vi "NonRobotDebugger.vi"() -> ()   [LabVIEW 2012]
uses:
  <vilib>/Utility/inputDevices.llb/joystickAcquire.vi
panel:
  out "Output Right":dbl(slide) scale=-1.0..1.0
  out "Output Left":dbl(slide) scale=-1.0..1.0
  out "X axis":dbl(slide) scale=-1.0..1.0
  out "Y axis":dbl(slide) scale=-1.0..1.0
  out "Throttle":dbl
  out "Steering":dbl
  out "Left Side Motors":dbl
  out "Right Side Motors":dbl
  in  "Gear":bool
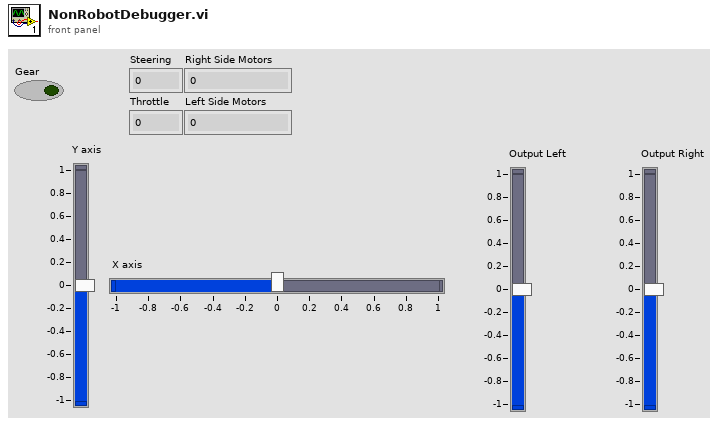
[diagram p1: front panel]
types:
  T1 = cluster{"X axis":i32, "Y axis":i32, "Z axis":i32, "X axis rotation":i32, "Y axis rotation":i32, "Z axis rotation":i32, "U axis":i32, "V axis":i32}
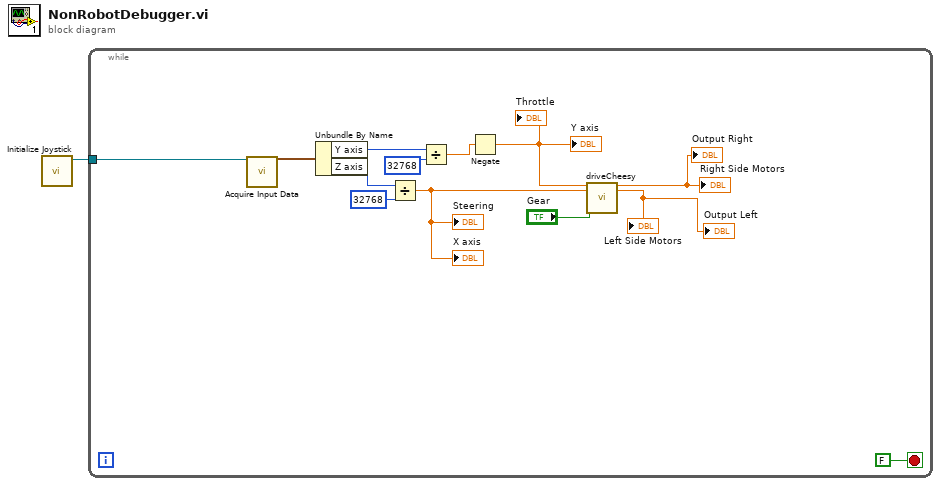
[diagram p0: block diagram]
diagram:
  n1 = call <vilib>:"Initialize Joystick.vi"() -> ("device ID"=w1:refnum<k1>)  [unwired: 10 in, 1 out]
  n2 = while {
    tunnel: w1 -> [w12]
    stop <- FALSE stop-if-true
    n3 = call-poly <vilib>:"Acquire Input Data.vi"("device ID"=w12) -> ("axis info"=w13:T1)  [unwired: 14 in, 4 out]
    n4 = Unbundle By Name(w13) -> ("Y axis"=w11:i32, "Z axis"=w9:i32)
    n5 = Divide(x=w9, y=32768) -> (x/y=w6:dbl)
    "Steering" <- w6
    "X axis" <- w6
    n6 = Divide(x=w11, y=32768) -> (x/y=w3:dbl)
    n7 = Negate(x=w3) -> (-x=w2:dbl)
    "Throttle" <- w2
    "Y axis" <- w2
    n8 = call "driveCheesy.vi"("Throttle"=w2, "Steering"=w6, "Gear"="Gear") -> ("Right Side Motors"=→"Right Side Motors" →"Output Right":dbl, "Left Side Motors"=→"Left Side Motors" →"Output Left":dbl)  [unwired: 15 in]
  }
